vi "DrawCurve.vi"(11 "曲线定义数组":string[](array[string])) -> (3 "曲线输出":cluster{"X":dbl[], "Y":dbl[]})   [LabVIEW 2020, in "Curve Editor.lvlib"]
uses:
  Curve Editor.lvlib
  Key Value/Key Value.lvlib
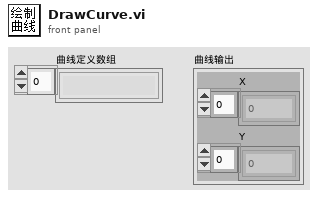
[diagram p1: front panel]
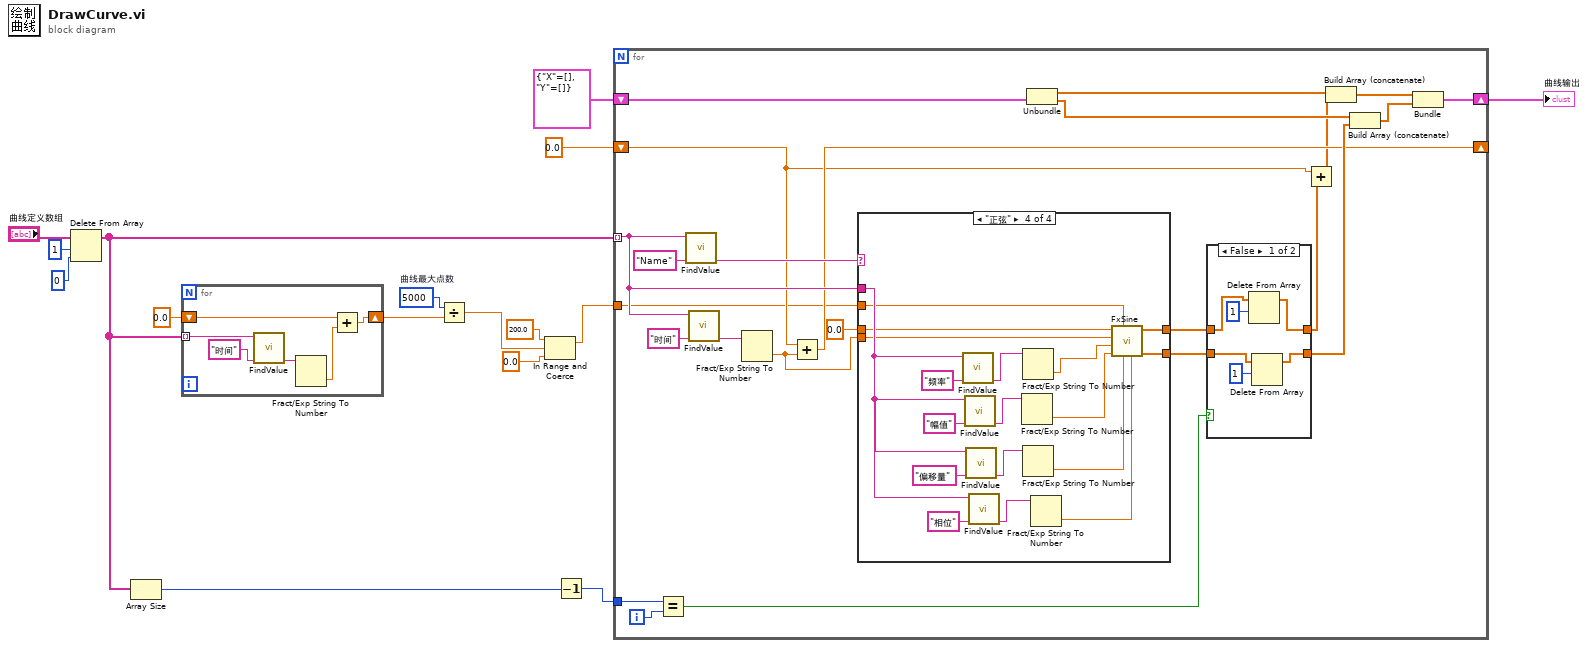
[diagram p0: block diagram]
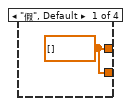
[diagram p3: hidden frame]
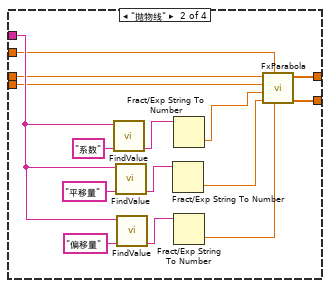
[diagram p4: hidden frame]
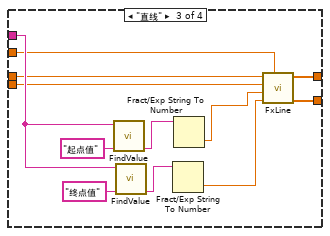
[diagram p5: hidden frame]
diagram:
  w6 = 5000  # 曲线最大点数
  n1 = Delete From Array(array="曲线定义数组", length=1 ("长度"), index=0 ("索引")) -> (array with subset deleted=w8:string[])  [unwired: 1 out]
  n2 = Array Size(array=w8) -> (size(s)=w12:i32)
  n3 = for {
    tunnel: w8 -> [w20] mode=indexing
    shift-right: [w18] -> w5
    shift-left: 0.0 -> [w17]
    n4 = call "FindValue.vi"("键"="时间", "键值串"=w20) -> ("值"=w22:string)  [unwired: 8 in, 1 out]
    n5 = Fract/Exp String To Number(string=w22) -> (number=w19:dbl)  [unwired: 3 in, 1 out]
    n6 = Add(x=w17, y=w19) -> (x+y=w18:dbl)
  }
  n7 = Divide(x=w6, y=w5) -> (x/y=w4:dbl)
  n8 = In Range and Coerce(upper limit=200.0, x=w4, lower limit=0.0) -> (coerced(x)=w1:dbl)  [unwired: 1 out]
  n9 = Decrement(x=w12) -> (x-1=w13:i32)
  n10 = for {
    tunnel: w8 -> [w31] mode=indexing
    tunnel: w13 -> [w43]
    shift-right: [w39] -> w15
    shift-left: cluster{"X":dbl[], "Y":dbl[]} {"X"=[], "Y"=[]} -> [w38]
    shift-right: [w28] -> _
    shift-left: 0.0 -> [w26]
    tunnel: w1 -> [w23]
    i -> [w44]
    n11 = Equal?(x=w43, y=w44) -> (x = y?=w42:bool)
    n12 = call "FindValue.vi"("键"="Name", "键值串"=w31) -> ("值"=w45:string)  [unwired: 8 in, 1 out]
    n13 = call "FindValue.vi"("键"="时间", "键值串"=w31) -> ("值"=w29:string)  [unwired: 8 in, 1 out]
    n14 = Fract/Exp String To Number(string=w29) -> (number=w25:dbl)  [unwired: 3 in, 1 out]
    n15 = Add(x=w26, y=w25) -> (x+y=w28:dbl)
    n16 = case shown="\"正弦\"" w45 {
      tunnel: w31 -> [_ w59 w74 w88]
      tunnel: [w55 w68 w80 w98] -> w41
      tunnel: [w55 w67 w79 w97] -> w40
      tunnel: w25 -> [_ w58 w72 w86]
      tunnel: 0.0 -> [_ w57 w73 w85]
      tunnel: w23 -> [_ w56 w71 w83]
      frame "假", Default {
        w55 = dbl[] [] ("X")
      }
      frame "抛物线" {
        n17 = call "FindValue.vi"("键"="系数", "键值串"=w59) -> ("值"=w60:string)  [unwired: 8 in, 1 out]
        n18 = call "FindValue.vi"("键"="平移量", "键值串"=w59) -> ("值"=w61:string)  [unwired: 8 in, 1 out]
        n19 = call "FindValue.vi"("键"="偏移量", "键值串"=w59) -> ("值"=w62:string)  [unwired: 8 in, 1 out]
        n20 = Fract/Exp String To Number(string=w61) -> (number=w69:dbl)  [unwired: 3 in, 1 out]
        n21 = Fract/Exp String To Number(string=w60) -> (number=w70:dbl)  [unwired: 3 in, 1 out]
        n22 = Fract/Exp String To Number(string=w62) -> (number=w66:dbl)  [unwired: 3 in, 1 out]
        n23 = call "FxParabola.vi"("偏移"=w66, "采样频率"=w56, "平移"=w69, "倍率"=w70, "终点时间"=w58, "起点时间"=w57) -> ("Y"=w67:dbl[], "X"=w68:dbl[])  [unwired: 4 in]
      }
      frame "直线" {
        n24 = call "FindValue.vi"("键"="起点值", "键值串"=w74) -> ("值"=w75:string)  [unwired: 8 in, 1 out]
        n25 = call "FindValue.vi"("键"="终点值", "键值串"=w74) -> ("值"=w76:string)  [unwired: 8 in, 1 out]
        n26 = Fract/Exp String To Number(string=w76) -> (number=w81:dbl)  [unwired: 3 in, 1 out]
        n27 = Fract/Exp String To Number(string=w75) -> (number=w82:dbl)  [unwired: 3 in, 1 out]
        n28 = call "FxLine.vi"("采样频率"=w71, "终点值"=w81, "起点值"=w82, "终点时间"=w72, "起点时间"=w73) -> ("Y"=w79:dbl[], "X"=w80:dbl[])  [unwired: 5 in]
      }
      frame "正弦" {
        n29 = call "FindValue.vi"("键"="频率", "键值串"=w88) -> ("值"=w90:string)  [unwired: 8 in, 1 out]
        n30 = call "FindValue.vi"("键"="幅值", "键值串"=w88) -> ("值"=w91:string)  [unwired: 8 in, 1 out]
        n31 = call "FindValue.vi"("键"="偏移量", "键值串"=w88) -> ("值"=w92:string)  [unwired: 8 in, 1 out]
        n32 = call "FindValue.vi"("键"="相位", "键值串"=w88) -> ("值"=w87:string)  [unwired: 8 in, 1 out]
        n33 = Fract/Exp String To Number(string=w91) -> (number=w99:dbl)  [unwired: 3 in, 1 out]
        n34 = Fract/Exp String To Number(string=w90) -> (number=w100:dbl)  [unwired: 3 in, 1 out]
        n35 = Fract/Exp String To Number(string=w92) -> (number=w96:dbl)  [unwired: 3 in, 1 out]
        n36 = Fract/Exp String To Number(string=w87) -> (number=w84:dbl)  [unwired: 3 in, 1 out]
        n37 = call "FxSine.vi"("相位"=w84, "偏移"=w96, "采样频率"=w83, "幅值"=w99, "频率"=w100, "终点时间"=w86, "起点时间"=w85) -> ("Y"=w97:dbl[], "X"=w98:dbl[])  [unwired: 3 in]
      }
    }
    n38 = Unbundle(w38) -> ("X"=w37:dbl[], "Y"=w35:dbl[])
    n39 = case shown="False" w42 {
      tunnel: w41 -> [w50 w54]
      tunnel: w40 -> [w48 w53]
      tunnel: [w49 w54] -> w36
      tunnel: [w47 w53] -> w34
      frame False {
        n40 = Delete From Array(array=w50, length=1 ("长度")) -> (array with subset deleted=w49:dbl[])  [unwired: 1 in, 1 out]
        n41 = Delete From Array(array=w48, length=1 ("长度")) -> (array with subset deleted=w47:dbl[])  [unwired: 1 in, 1 out]
      }
      frame True {
      }
    }
    n42 = Add(x=w26, y=w36) -> (x+y=w27:dbl[])
    n43 = Build Array (concatenate)(w37, w27) -> (w33:dbl[])
    n44 = Build Array (concatenate)(w35, w34) -> (w32:dbl[])
    n45 = Bundle(w33, w32) -> (w39:cluster{dbl[], dbl[]})  [unwired: 1 in]
  }
  "曲线输出" <- w15
